vi "TVA (SubVI).vi"(6 "sim/sens rotation param (rates/angles)":dbl[][](array[numeric]), 9 "Initial Param":T1, 10 "sim_running":bool, 11 "Output Control":dbl[](array[numeric])) -> (3 "act_b":T2)   [LabVIEW 2017]
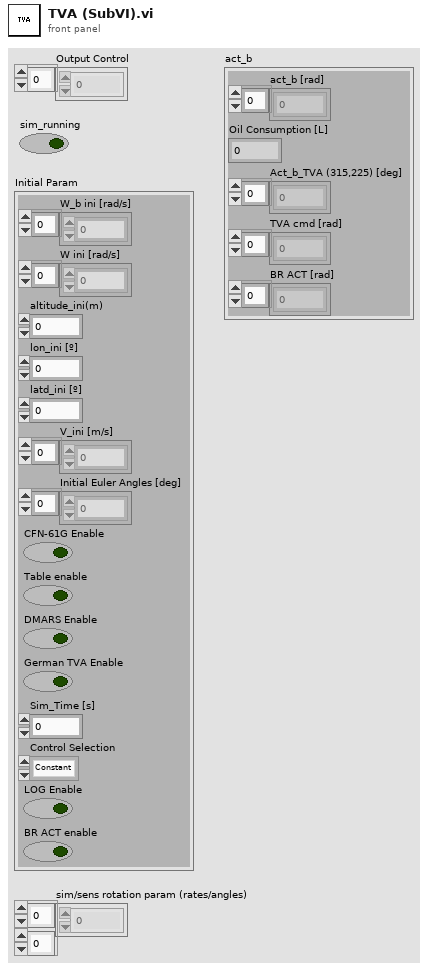
[diagram p1: front panel]
types:
  T1 = cluster{"W_b ini [rad/s]":dbl[], "W ini [rad/s]":dbl[], "altitude_ini(m)":dbl, "lon_ini [º]":dbl, "latd_ini [º]":dbl, "V_ini [m/s]":dbl[], "Initial Euler Angles [deg]":dbl[], "CFN-61G Enable":bool, "Table enable":bool, "DMARS Enable":bool, "German TVA Enable":bool, "Sim_Time [s]":dbl, "Control Selection":enum16{"Constant", "TVA E-BOX", "Sim Control"}, "LOG Enable":bool, "BR ACT enable":bool}
  T2 = cluster{"act_b [rad]":dbl[], "Oil Consumption [L]":dbl, "Act_b_TVA (315,225) [deg]":dbl[], "TVA cmd [rad]":dbl[], "BR ACT [rad]":dbl[]}
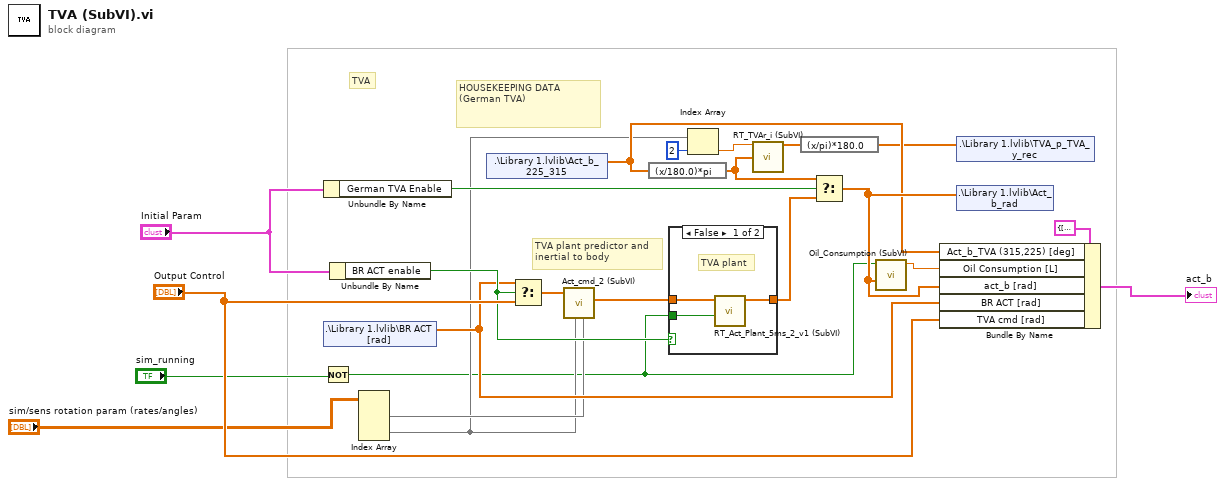
[diagram p0: block diagram]
diagram:
  # "TVA plant predictor and\ninertial to body"
  # "HOUSEKEEPING DATA (German TVA)"
  # "TVA"
  n1 = Not(x="sim_running") -> (.not. x?=w7:bool)
  n2 = Unbundle By Name("Initial Param") -> ("German TVA Enable"=w15:bool)
  n3 = shared-variable ".\\Library 1.lvlib\\BR ACT [rad]"() -> (w17:dbl[])  [unwired: 1 in, 1 out]
  n4 = Unbundle By Name("Initial Param") -> ("BR ACT enable"=w18:bool)
  n5 = Index Array(array="sim/sens rotation param (rates/angles)") -> (element #1=w13:dbl[], element #2=w8:dbl[])  [unwired: 4 in]
  n6 = shared-variable ".\\Library 1.lvlib\\Act_b_225_315"() -> (w12:dbl[])  [unwired: 1 in, 1 out]
  n7 = Select(t=w17, s=w18, f="Output Control") -> (s? t:f=w20:dbl[])
  n8 = call "Act_cmd_2 (SubVI).vi"("W_b [rad/s]"=w13, "Euler Angles [rad]"=w8, "TVA_cmd [rad]"=w20) -> ("Act315_Act225"=w22:dbl[])  [unwired: 7 in, 1 out]
  n9 = expression code="(x/180.0)*pi" ("degrees to radians")(w12) -> (w6:dbl[])
  n10 = case shown="False" w18 {
    tunnel: [w26 w27] -> w21
    tunnel: w22 -> [w24 w27]
    tunnel: w7 -> [w25 _]
    frame False {
      # "TVA plant"
      n11 = call "RT_Act_Plant_5ms_2_v1 (SubVI).vi"("not.Sim_Running"=w25, "TVA_cmd"=w24) -> ("Act_b"=w26:dbl[])  [unwired: 7 in, 2 out]
    }
    frame True {
    }
  }
  n12 = Index Array(array=w8, index=2) -> (element=w4:dbl)
  n13 = call "RT_TVAr_i (SubVI).vi"("roll1"=w4, "Act315_Act225"=w6) -> ("TVA_p/TVA_y"=w5:dbl[])  [unwired: 13 in]
  n14 = expression code="(x/pi)*180.0" ("radians to degrees")(w5) -> (w2:dbl[])
  n15 = Select(t=w6, s=w15, f=w21) -> (s? t:f=w16:dbl[])
  n16 = call "Oil_Consumption (SubVI).vi"("act_b"=w16, "not.Sim_Running"=w7) -> ("Oil Consumption [L]"=w11:dbl)  [unwired: 9 in]
  n17 = Bundle By Name(cluster=T2 {"act_b [rad]"=[], "Oil Consumption [L]"=0.0, "Act_b_TVA (315,225) [deg]"=[], "TVA cmd [rad]"=[], "BR ACT [rad]"=[]} ("TVA"), "Act_b_TVA (315,225) [deg]"=w12, "Oil Consumption [L]"=w11, "act_b [rad]"=w16, "BR ACT [rad]"=w17, "TVA cmd [rad]"="Output Control") -> (→"act_b":T2)
  n18 = shared-variable ".\\Library 1.lvlib\\TVA_p_TVA_y_rec"(w2) -> ()  [unwired: 1 in, 1 out]
  n19 = shared-variable ".\\Library 1.lvlib\\Act_b_rad"(w16) -> ()  [unwired: 1 in, 1 out]
